vi "CMD_Global.vi"() -> ()   [LabVIEW 2017]
panel:
  in  "CMD_TEST Axis":dbl
  in  "CMD_TEST BUTTON":bool
  # "The Names of the Data items in the Global Variable MUST describe who the Single Writer is\nNaming Convention of all Data Items is:   \nCMD_Data Name\nExamples:\nCMD_Drive Data"
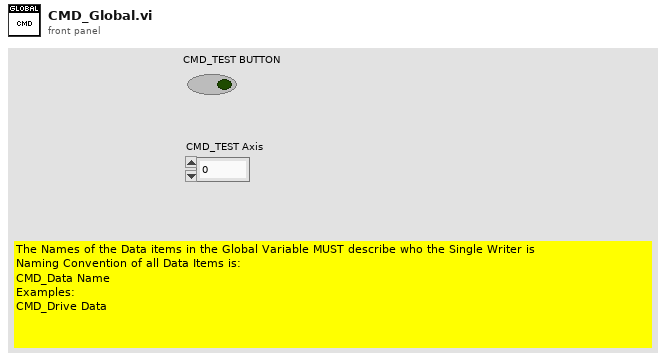
[diagram p1: front panel]
diagram:
